vi "Actuators Set Acceleration.vi"(0 "Notifier Name":string, 5 "Channel":i32[](array[numeric]), 7 "Acceleration":dbl[](array[numeric]), 11 "Error In":errorcluster) -> (4 "Notifier Name Out":string, 15 "Error Out":errorcluster)   [LabVIEW 2020]
uses:
  Actuators Controls/Actuators Note Type.ctl
  Actuators Controls/Actuators Actions.ctl
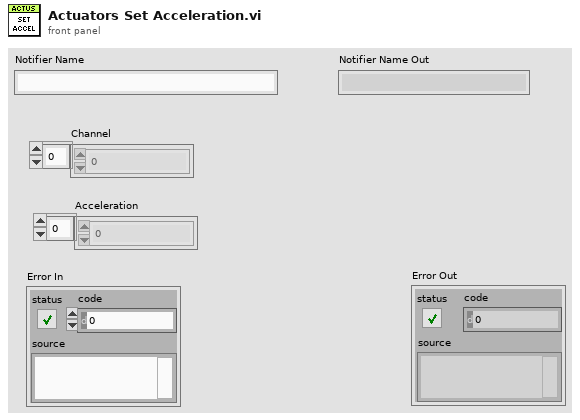
[diagram p1: front panel]
types:
  T1 = typedef "Actuators Note Type.ctl" = cluster{"Actions":T2, "Cmd Received ":bool, "Setpoint":dbl[], "Position":dbl[], "Channel":i32[], "Jog Step":dbl[], "Velocity":dbl[], "Acceleration":dbl[], "Status Bits":u32[], "Moving":bool[]}
  T2 = typedef "Actuators Actions.ctl" = enum16{"Nothing", "Get Position", "Get Acceleration", "Get Velocity", "Get Jog Step", "Set Acceleration", "Set Velocity", "Set Jog Step", "Move Absolute", "Move Relative", "Jog Forward", "Jog Reverse", "Set Moving", "Halt", "Quit"}
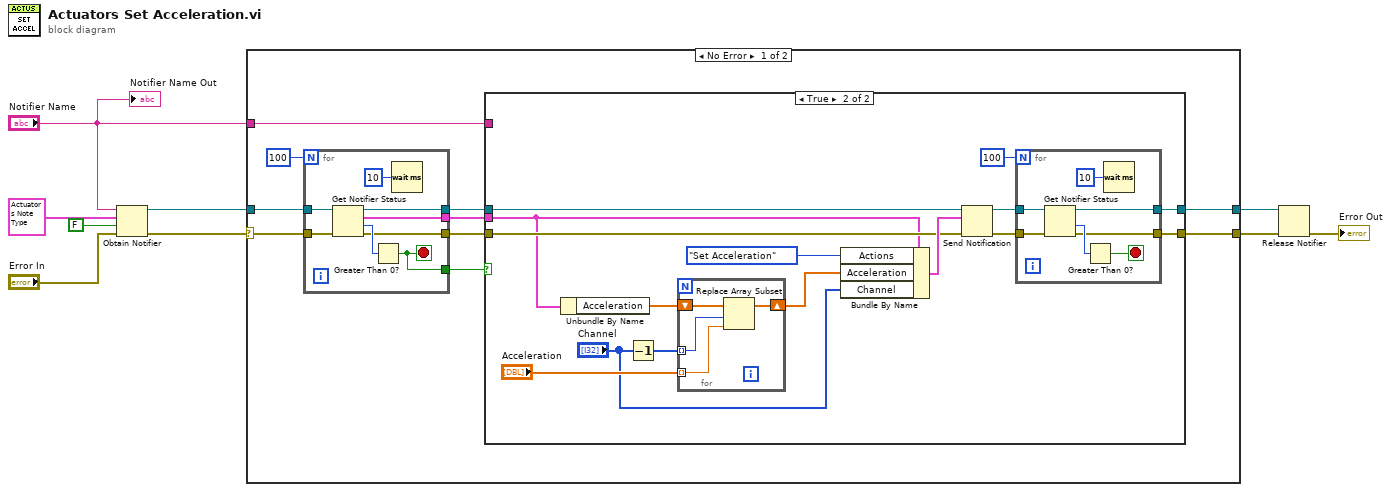
[diagram p0: block diagram]
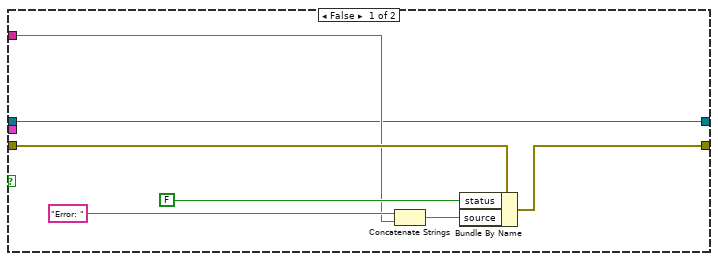
[diagram p2: hidden frame]
diagram:
  n1 = Obtain Notifier(name (unnamed)="Notifier Name", notification data type=T1 {"Actions"=enum."Nothing", "Cmd Received "=FALSE, "Setpoint"=[], "Position"=[], "Channel"=[], "Jog Step"=[], "Velocity"=[], "Acceleration"=[], "Status Bits"=[], "Moving"=[]} ("Actuators Note"), create if not found? (T)=FALSE, error in (no error)="Error In") -> (notifier out=w5:refnum<notifier>, error out=w8:errorcluster)  [unwired: 1 out]
  n2 = case shown="No Error" w8 {
    selector: w8 -> [w17 w61]
    tunnel: w5 -> [w18 w62]
    tunnel: "Notifier Name" -> [w12 _]
    tunnel: [w11 w62] -> w4
    tunnel: [w10 w61] -> w3
    frame No Error {
      n3 = for {
        N: 100 -> [_]
        tunnel: [w59] -> w14
        tunnel: w18 -> [w60]
        tunnel: [w58] -> w15
        tunnel: w17 -> [w55]
        tunnel: [w54] -> w16
        tunnel: [w53] -> w13
        stop <- w54 stop-if-true
        n4 = Get Notifier Status(notifier=w60, error in (no error)=w55) -> (notifier out=w58:refnum<notifier>, current notification=w59:T1, # waiting=w57:i32, error out=w53:errorcluster)  [unwired: 1 out]
        n5 = Greater Than 0?(x=w57) -> (x > 0?=w54:bool)
        n6 = Wait (ms)(milliseconds to wait=u32 10) -> ()  [unwired: 1 out]
      }
      n7 = case shown="True" w16 {
        tunnel: w15 -> [w21 w41]
        tunnel: w14 -> [_ w32]
        tunnel: w13 -> [w26 w38]
        tunnel: w12 -> [w22 _]
        tunnel: [w21 w33] -> w11
        tunnel: [w20 w34] -> w10
        frame False {
          n8 = Concatenate Strings("Error: " ("source"), w22) -> (w23:string)
          n9 = Bundle By Name(cluster=w26, "status"=FALSE, "source"=w23) -> (w20:errorcluster)
        }
        frame True {
          n10 = Unbundle By Name(w32) -> ("Acceleration"=w30:dbl[])
          n11 = Decrement(x="Channel") -> (x-1=w27:i32[])
          n12 = for {
            tunnel: w27 -> [w45] mode=indexing
            tunnel: "Acceleration" -> [w44] mode=indexing
            shift-right: [w42] -> w29
            shift-left: w30 -> [w43]
            n13 = Replace Array Subset(array=w43, new element=w44, index=w45) -> (w42:dbl[])
          }
          n14 = Bundle By Name(cluster=w32, "Actions"=Actuators_Actions."Set Acceleration", "Acceleration"=w29, "Channel"="Channel") -> (w39:T1)
          n15 = Send Notification(notification=w39, notifier=w41, error in (no error)=w38) -> (notifier out=w36:refnum<notifier>, error out=w35:errorcluster)
          n16 = for {
            N: 100 -> [_]
            tunnel: w36 -> [w52]
            tunnel: [w51] -> w33
            tunnel: w35 -> [w48]
            tunnel: [w46] -> w34
            stop <- w47 stop-if-true
            n17 = Get Notifier Status(notifier=w52, error in (no error)=w48) -> (notifier out=w51:refnum<notifier>, # waiting=w50:i32, error out=w46:errorcluster)  [unwired: 2 out]
            n18 = Greater Than 0?(x=w50) -> (x > 0?=w47:bool)
            n19 = Wait (ms)(milliseconds to wait=u32 10) -> ()  [unwired: 1 out]
          }
        }
      }
    }
    frame Error {
    }
  }
  n20 = Release Notifier(notifier=w4, error in (no error)=w3) -> (error out=→"Error Out":errorcluster)  [unwired: 1 in, 2 out]
  "Notifier Name Out" <- "Notifier Name"
